vi "Create Default Scaffold INI.vi"(8 "error in (no error)":errorcluster) -> (0 "error out":errorcluster)   [LabVIEW 2020, in "Negentropic IDE.lvlib"]
uses:
  <resource>/Framework/Providers/Negentropic IDE/Negentropic IDE/Negentropic IDE.lvlib
  <resource>/Framework/Providers/Negentropic IDE/Negentropic IDE/Folder Config.ctl
  <resource>/Framework/Providers/Negentropic IDE/Negentropic IDE/Scope.ctl
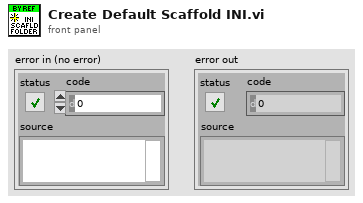
[diagram p1: front panel]
types:
  T1 = typedef "Negentropic IDE.lvlib/Folder Config.ctl" = cluster{"Path":string, "Scope":T2}
  T2 = typedef "Negentropic IDE.lvlib/Scope.ctl" = enum32{"invalid scope", "public", "private", "protected", "community"}
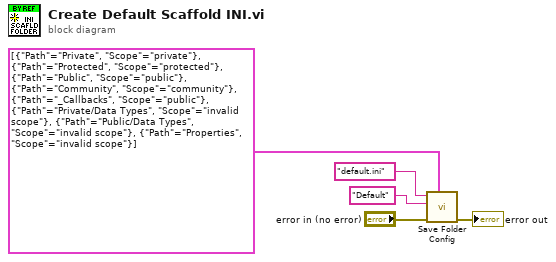
[diagram p0: block diagram]
diagram:
  n1 = call <resource>:"Save Folder Config.vi"("Folder Config"=T1[] [{"Path"="Private", "Scope"=enum."private"}, {"Path"="Protected", "Scope"=enum."protected"}, {"Path"="Public", "Scope"=enum."public"}, {"Path"="Community", "Scope"=enum."community"}, {"Path"="_Callbacks", "Scope"=enum."public"}, {"Path"="Private/Data Types", "Scope"=enum."invalid scope"}, {"Path"="Public/Data Types", "Scope"=enum."invalid scope"}, {"Path"="Properties", "Scope"=enum."invalid scope"}], "error in (no error)"="error in (no error)", "Name"="Default" ("key"), "INI Filename"="default.ini" ("name or relative path")) -> ("error out"=→"error out":errorcluster)  [unwired: 7 in]
